vi "proj_sim_my_MATLAB.vi"() -> ()   [LabVIEW 2023]
uses:
  <vilib>/addons/Modulation/Analog/support/mod_Set Error Source.vi
  <vilib>/addons/Modulation/Digital/Support/Common/Validators/mod_AWGN Validate.vi
  <vilib>/addons/Modulation/Digital/Impairments/subVIs/mod_createSeeds.vi
  <vilib>/addons/Modulation/Digital/Support/Common/Validators/mod_Validate Samples Per Symbol.vi
  <vilib>/addons/Modulation/Analog/support/Validators/mod_Validate Complex Waveform.vi
  <vilib>/addons/Modulation/Analog/support/Validators/mod_WFErrorHandler.vi
  <vilib>/addons/Modulation/Digital/Support/Common/Validators/mod_Generate Filter Coefficients Validate.vi
  <vilib>/addons/Modulation/Digital/General/subVIs/mod_Generate Filter Coefficients.vi
  <vilib>/addons/Modulation/Digital/General/MT Generate QAM System Parameters(M).vi
  <vilib>/addons/Modulation/Digital/General/subVIs/mod_Generate Bits PN Sequence.vi
  <vilib>/Analysis/1siggen.llb/Gaussian White Noise (obs 90).vi
  <vilib>/addons/Modulation/Analog/MT Upconvert Baseband (Complex).vi
  <vilib>/addons/Modulation/Analog/MT Downconvert Passband (Complex).vi
  <vilib>/addons/Modulation/niDMT.lvlib
  <vilib>/addons/Modulation/niAMT.lvlib
panel:
  out "?":T1 {"oversampled data" format="%.2f"; "constellation" format="%.2f"}
  out "dt":dbl
  out "Mod Up Const":T2(graph)
  out "constellation graph 4":T2(array[cluster]) {"oversampled data" format="%.2f"; "constellation" format="%.2f"}
  out "size(s) 3":i32
  out "size(s) 2":i32
  out "bits per symbol":i32
  in  "pulse shaping filter (none)":T3(ring)
  out "In-phase component":cluster{"t0":dbl, "dt":dbl, "Y":dbl[]}(graph)
  out "Quadrature component":cluster{"t0":dbl, "dt":dbl, "Y":dbl[]}(graph)
  out "Mod Constellation":T2(graph)
  in  "M-QAM (16)":i32=16
  in  "Eb/N0 (10 dB)":dbl=10.0 format="%.2f"
  out "Demodulated":cluster{"t0":dbl, "dt":dbl, "Y":dbl[]}(graph)
  out "Modulated":cluster{"t0":dbl, "dt":dbl, "Y":dbl[]}(graph)
  in  "carrier frequency (Hz)":dbl min=-0.5 max=0.5 format="%.2f"
  in  "passband bandwidth (Hz)":dbl format="%.2p"
  in  "advanced filter parameters":T4={"passband ripple (dB)"=0.01, "stopband start (Hz)"=0.0, "stopband gain (dB)"=-96.0, "compute filter stopband ? (T)"=TRUE}
  in  "pulse shaping samples per symbol (16)":i32=16
  in  "matched samples per symbol (16)":i32=16
  in  "filter parameter":dbl=0.5 format="%.2f"
  in  "samples per symbol (16)":i32=16
  in  "symbol rate (Hz)":dbl=1.0 format="%.2f"
  in  "stop":bool
  out "Demod Const Down":T2(graph)
  out "constellation graph 2":T2(array[cluster]) {"oversampled data" format="%.2f"; "constellation" format="%.2f"}
  out "Demod Const 2":T2(graph)
  out "constellation graph 3":T2(array[cluster]) {"oversampled data" format="%.2f"; "constellation" format="%.2f"}
  out "size(s)":i32
  out "1-D Array of Real":dbl[](array[numeric])
  out "Input":waveform(dbl)(graph)
  in  "path":path
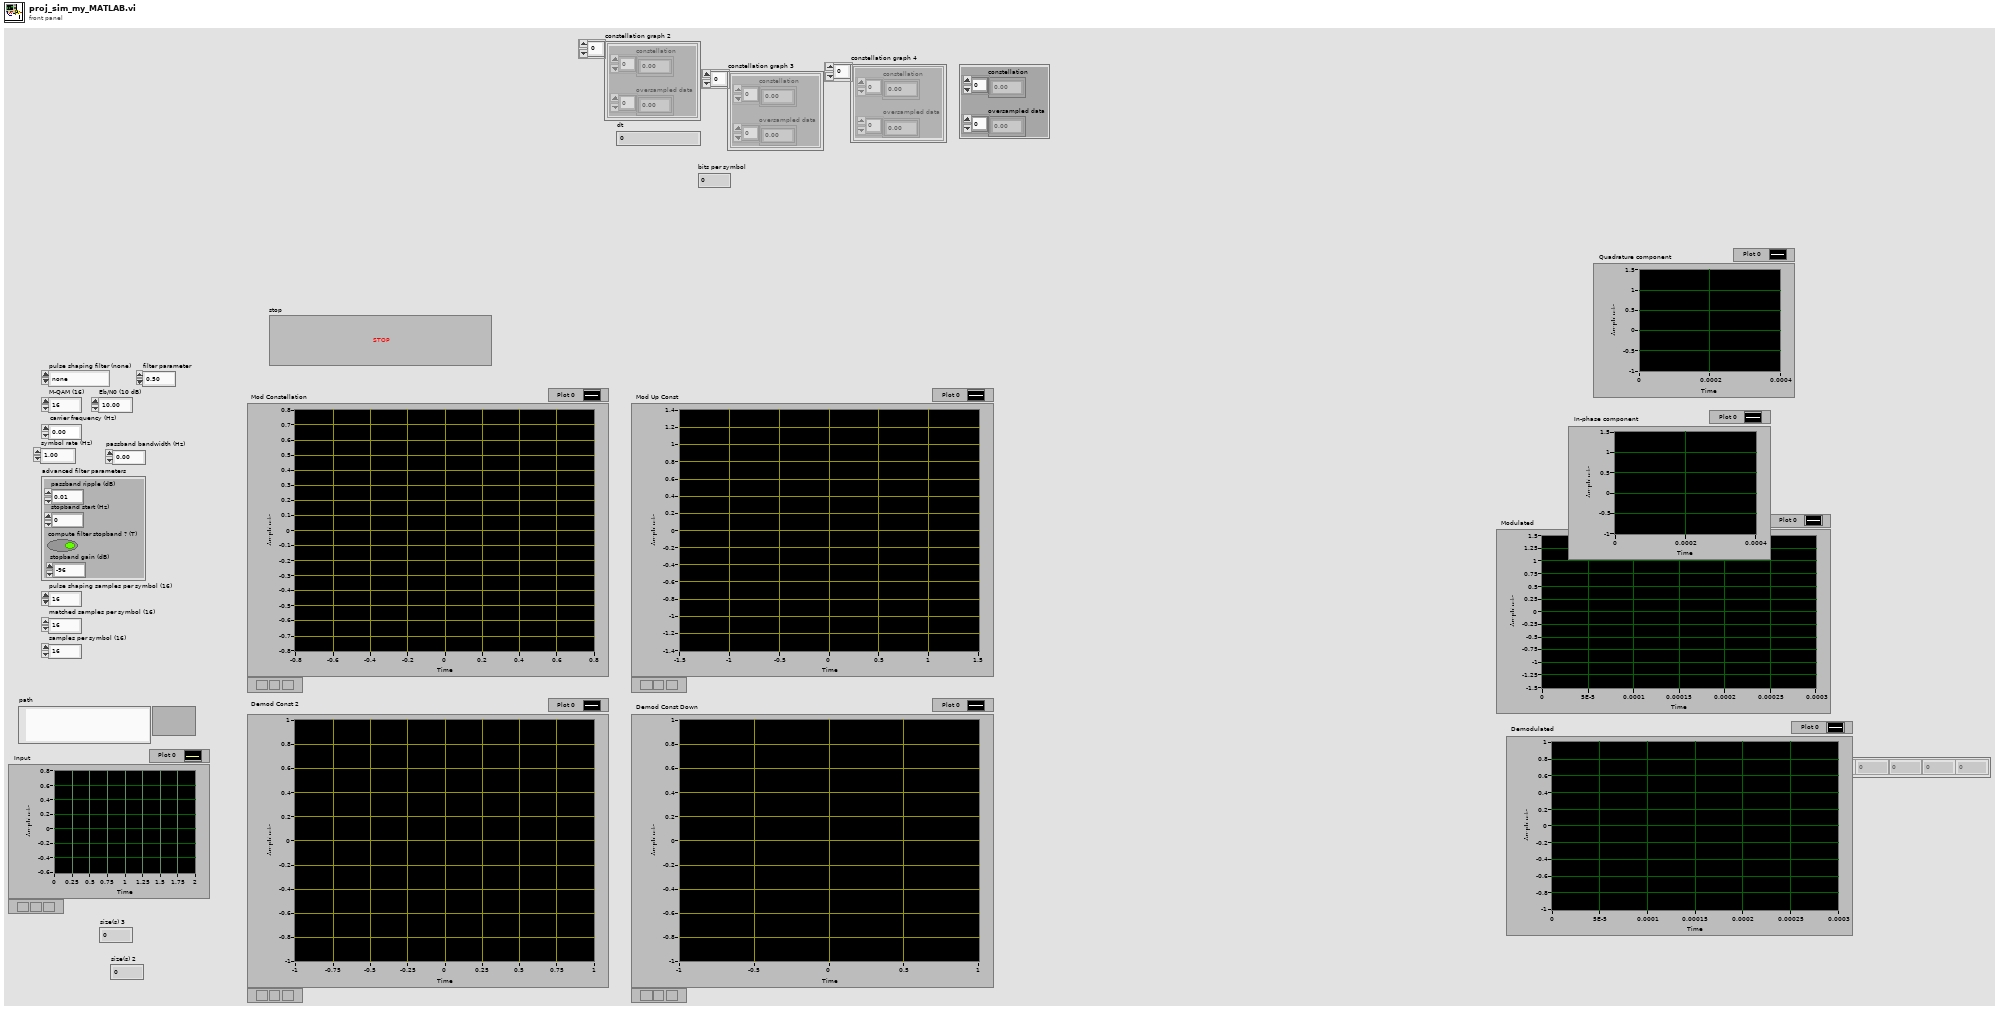
[diagram p1: front panel]
types:
  T1 = cluster{"constellation":dbl[], "oversampled data":dbl[]}
  T2 = cluster{"constellation":dbl[], "oversampled data":dbl[]}[]
  T3 = enum16{"none", "Raised Cosine", "Root Raised Cos", "Gaussian"}
  T4 = cluster{"passband ripple (dB)":dbl, "stopband start (Hz)":dbl, "stopband gain (dB)":dbl, "compute filter stopband ? (T)":bool}
  T5 = enum16{"FSK", "PSK", "QAM", "MSK", "PAM", "ASK", "CPM"}
  T6 = cluster{"samples per symbol (16)":i32, "symbol map":cdb[]}
  T7 = typedef "niAMT.lvlib/Complex Data Waveform.ctl" = cluster{"t0":dbl, "dt":dbl, "Y":cdb[]}
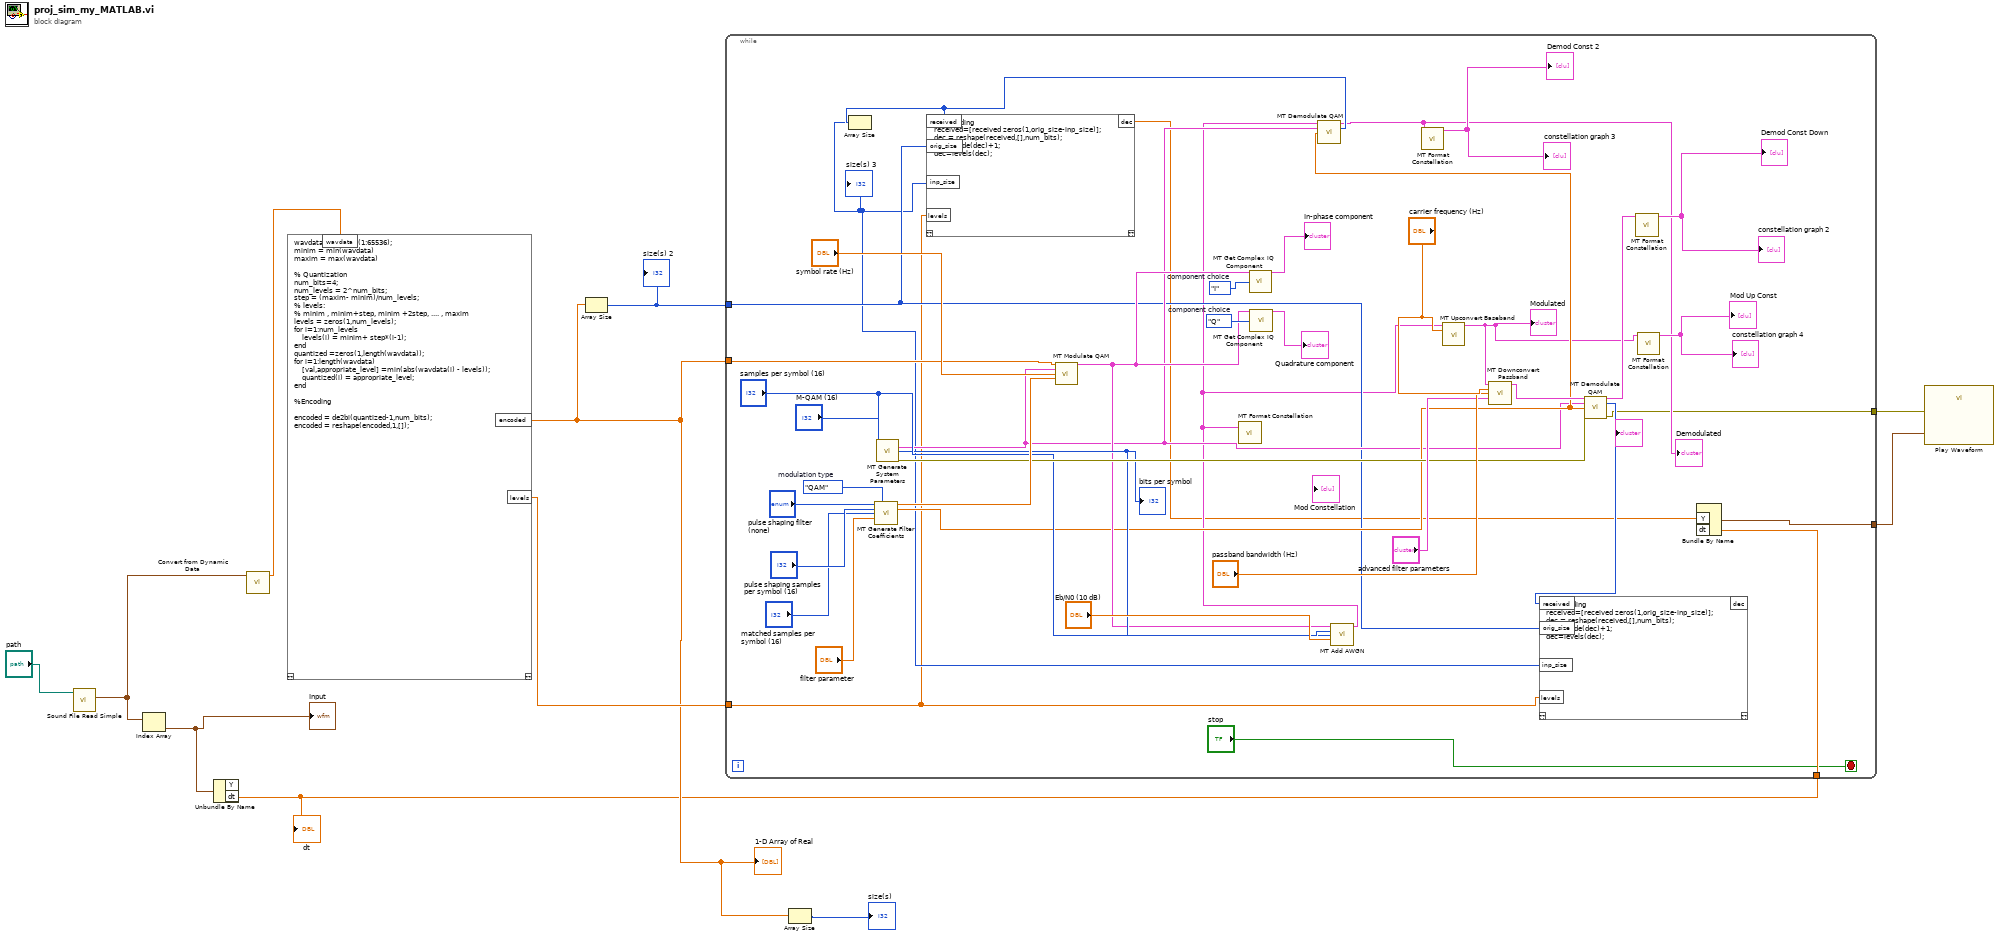
[diagram p0: block diagram]
diagram:
  n1 = call <vilib>:"Sound File Read Simple.vi"("path"="path") -> ("data"=w6:waveform(dbl)[])  [unwired: 7 in, 3 out]
  n2 = Index Array "Index Array"(array=w6) -> (element=w8:waveform(dbl))  [unwired: 1 in]
  "Input" <- w8
  n3 = Unbundle By Name(w8) -> ("dt"=w3:dbl)  [unwired: 1 out]
  "dt" <- w3
  n4 = call "Convert from Dynamic Data"("Dynamic Data Type"=w6) -> ("Array"=w10:dbl[])  [unwired: 3 in]
  n5 = script code="wavdata=wavdata(1:65536);\nminim = min(wavdata)\nmaxim = max(wavdata)\n\n% Quantization\nnum_bits=4;\nnum_levels = 2^num_bits;\nstep = (maxim- minim)/num_levels;\n% levels:\n% minim , minim+step, minim +2step, .... , maxim\nlevels = zeros(1,num_levels);\nfor i=1:num_levels\n    levels(i) = minim+ step*(i-1);\nend\nquantized =zeros(1,length(wavdata));\nfor i=1:length(wavdata)\n    [val,appropriate_level] =min(abs(wavdata(i) - levels));\n    quantized(i) = appropriate_level;\nend\n\n%Encoding\n\nencoded = de2bi(quantized-1,num_bits);\nencoded = reshape(encoded,1,[]);"("wavdata"=w10) -> ("encoded"=w5:dbl[], "levels"=w9:dbl[])  [unwired: 1 in, 1 out]
  "1-D Array of Real" <- w5
  n6 = Array Size(array=w5) -> (size(s)=w4:i32)
  "size(s) 2" <- w4
  n7 = while {
    tunnel: w9 -> [w16]
    tunnel: w3 -> [w37]
    tunnel: w5 -> [w24]
    tunnel: w4 -> [w18]
    tunnel: [w12] -> w2
    tunnel: [w13] -> w1
    stop <- "stop" stop-if-true
    w49 = enum16{"I", "Q", "Magnitude", "Phase"}."Q"  # component choice
    w50 = enum16{"I", "Q", "Magnitude", "Phase"}."I"  # component choice
    w52 = T5."QAM"  # modulation type
    n8 = call <vilib>:"MT Generate Filter Coefficients.vi"("pulse shaping filter (none)"="pulse shaping filter (none)", "modulation type"=w52, "pulse shaping samples per symbol (16)"="pulse shaping samples per symbol (16)", "matched samples per symbol (16)"="matched samples per symbol (16)", "filter parameter"="filter parameter") -> ("pulse shaping filter coefficients"=w47:dbl[], "matched filter coefficients"=w26:dbl[])  [unwired: 8 in, 1 out]
    n9 = call-poly <vilib>:"MT Generate System Parameters.vi"("samples per symbol (16)"="samples per symbol (16)", "M-QAM (16)"="M-QAM (16)") -> ("QAM system parameters"=w25:T6, "bits per symbol"=w32:i32, "error out"=w36:errorcluster)  [unwired: 11 in]
    "bits per symbol" <- w32
    n10 = call <vilib>:"MT Modulate QAM.vi"("input bit stream"=w24, "QAM system parameters"=w25, "symbol rate (Hz)"="symbol rate (Hz)", "pulse shaping filter coefficients"=w47) -> ("output complex waveform"=w28:T7)  [unwired: 9 in, 2 out]
    n11 = call <vilib>:"MT Get Complex IQ Component.vi"("IQ data (complex) in"=w28, "component choice"=w50) -> ("IQ data (complex) out"=→"In-phase component":cluster{"t0":dbl, "dt":dbl, "Y":cdb[]})  [unwired: 11 in, 2 out]
    n12 = call <vilib>:"MT Get Complex IQ Component.vi"("IQ data (complex) in"=w28, "component choice"=w49) -> ("IQ data (complex) out"=→"Quadrature component":cluster{"t0":dbl, "dt":dbl, "Y":cdb[]})  [unwired: 11 in, 2 out]
    n13 = call <vilib>:"MT Add AWGN.vi"("input complex waveform"=w28, "samples per symbol (16)"="samples per symbol (16)", "bits per symbol (1)"=w32, "Eb/N0 (10 dB)"="Eb/N0 (10 dB)") -> ("output complex waveform"=w15:T7)  [unwired: 9 in, 2 out]
    n14 = call <vilib>:"MT Format Constellation.vi"("waveform"=w15) -> ()  [unwired: 13 in, 2 out]
    n15 = call <vilib>:"MT Demodulate QAM.vi"("input complex waveform"=w15, "QAM system parameters"=w25, "matched filter coefficients"=w26) -> ("recovered complex waveform"=w20:T7, "output bit stream"=w23:i8[])  [unwired: 8 in, 3 out]
    "Demodulated" <- w20
    n16 = Array Size(array=w23) -> (size(s)=w17:i32)
    "size(s) 3" <- w17
    n17 = script code="% Decoding \nreceived=[received zeros(1,orig_size-inp_size)];\ndec = reshape(received,[],num_bits);\ndec=bi2de(dec)+1;\ndec=levels(dec);"("received"=w23, "levels"=w16, "inp_size"=w17, "orig_size"=w18) -> ("dec"=w14:dbl[])  [unwired: 1 in, 1 out]
    n18 = call <vilib>:"MT Format Constellation.vi"("waveform"=w20) -> ("constellation graph"=→"Demod Const 2" →"constellation graph 3":T2)  [unwired: 13 in, 1 out]
    n19 = call-poly <vilib>:"MT Upconvert Baseband.vi"("complex waveform"=w15, "carrier frequency (Hz)"="carrier frequency (Hz)") -> ("upconverted waveform (complex)"=w21:T7)  [unwired: 12 in, 1 out]
    "Modulated" <- w21
    n20 = call-poly <vilib>:"MT Downconvert Passband.vi"("complex waveform"=w21, "carrier frequency (Hz)"="carrier frequency (Hz)", "passband bandwidth (Hz)"="passband bandwidth (Hz)", "advanced filter parameters"="advanced filter parameters") -> ("downconverted waveform (complex)"=w44:T7)  [unwired: 8 in, 3 out]
    n21 = call <vilib>:"MT Demodulate QAM.vi"("input complex waveform"=w44, "QAM system parameters"=w25, "matched filter coefficients"=w26, "error in (no error)"=w36) -> ("recovered complex waveform"=w30:T7, "output bit stream"=w19:i8[], "error out"=w13:errorcluster)  [unwired: 7 in, 2 out]
    n22 = script code="% Decoding \nreceived=[received zeros(1,orig_size-inp_size)];\ndec = reshape(received,[],num_bits);\ndec=bi2de(dec)+1;\ndec=levels(dec);"("received"=w19, "levels"=w16, "inp_size"=w17, "orig_size"=w18) -> ()  [unwired: 1 in, 2 out]
    n23 = call <vilib>:"MT Format Constellation.vi"("waveform"=w30) -> ("constellation graph"=→"Demod Const Down" →"constellation graph 2":T2)  [unwired: 13 in, 1 out]
    n24 = call <vilib>:"MT Format Constellation.vi"("waveform"=w21) -> ("constellation graph"=→"Mod Up Const" →"constellation graph 4":T2)  [unwired: 13 in, 1 out]
    n25 = Bundle By Name("Y"=w14, "dt"=w37) -> (w12:waveform(dbl))  [unwired: 1 in]
  }
  n26 = Array Size(array=w5) -> (size(s)=→"size(s)":i32)
  n27 = call "Play Waveform"("Data"=w2, "error in"=w1) -> ()  [unwired: 17 in, 1 out]
